vi "Write PWM Lengths.vi"(8 "error in (no error)":errorcluster, 10 "PWM Lengths":dbl[unit][](array[numeric]) format="%.1g", 11 "Set Lengths Msg in":refnum<class "Set Lengths Msg.lvclass">) -> (0 "error out":errorcluster, 3 "Set Lengths Msg out":refnum<class "Set Lengths Msg.lvclass">)   [LabVIEW 2020, in "BNT_ULx.lvlib" / "Set Lengths Msg.lvclass"]
uses:
  Set Lengths Msg.lvclass
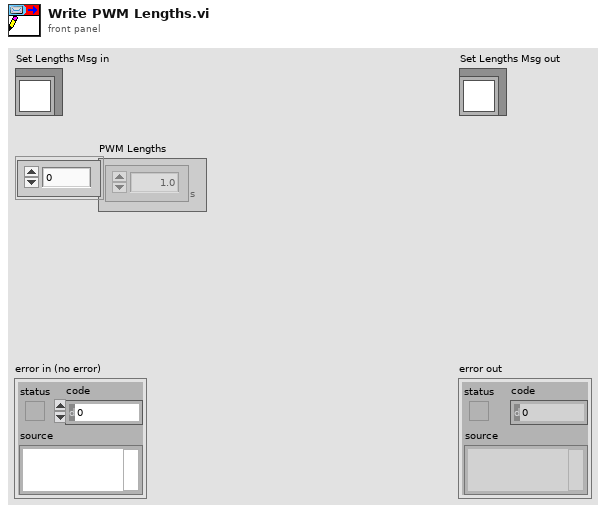
[diagram p1: front panel]
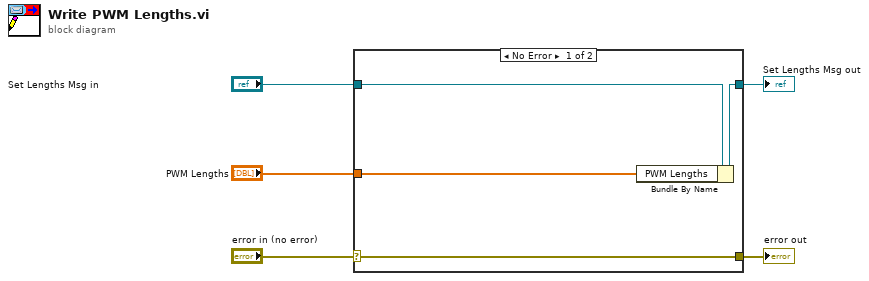
[diagram p0: block diagram]
diagram:
  n1 = case shown="No Error" "error in (no error)" {
    selector: "error in (no error)" -> [w9 w10]
    tunnel: [w9 w10] -> w4
    tunnel: [w7 w11] -> w2
    tunnel: "Set Lengths Msg in" -> [w8 w11]
    tunnel: "PWM Lengths" -> [w6 _]
    frame No Error {
      n2 = Bundle By Name(cluster=w8, "PWM Lengths"=w6) -> (w7:refnum<class "Set Lengths Msg.lvclass">)
    }
    frame Error {
    }
  }
  "error out" <- w4
  "Set Lengths Msg out" <- w2
